vi "Tree.vi"   [LabVIEW 2016, in "LV to ITX.lvclass"]
uses:
  LV to ITX.lvclass
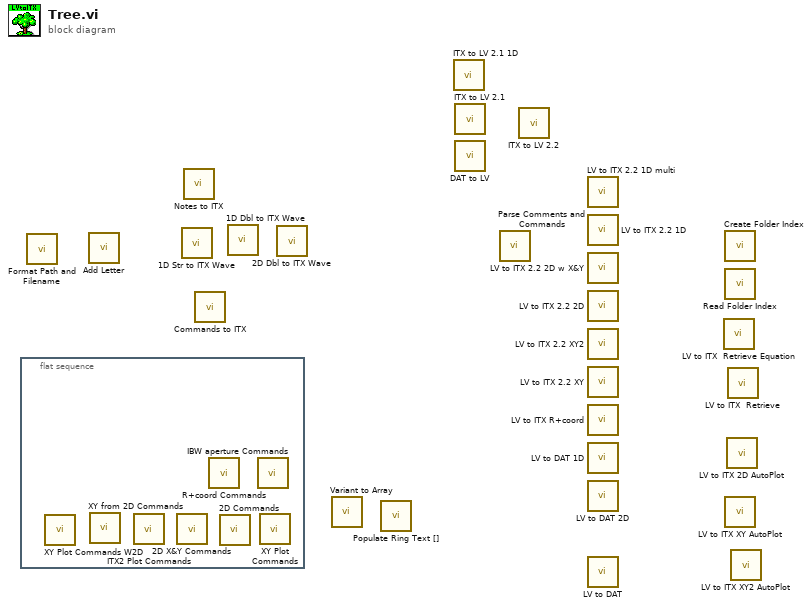
[diagram p0: block diagram]
diagram:
  n1 = flat-sequence {
    frame #0 {
      n2 = call "XY Plot Commands W2D.vi"() -> ()  [unwired: 5 in, 1 out]
      n3 = call "XY from 2D Commands.vi"() -> ()  [unwired: 2 in, 1 out]
      n4 = call "ITX2 Plot Commands.vi"() -> ()  [unwired: 6 in, 1 out]
      n5 = call "2D X&Y Commands.vi"() -> ()  [unwired: 10 in, 2 out]
      n6 = call "R+coord Commands.vi"() -> ()  [unwired: 15 in, 1 out]
      n7 = call "2D Commands.vi"() -> ()  [unwired: 15 in, 1 out]
      n8 = call "IBW aperture Commands.vi"() -> ()  [unwired: 4 in, 1 out]
      n9 = call "XY Plot Commands.vi"() -> ()  [unwired: 6 in, 1 out]
    }
  }
  n10 = call "Format Path and Filename.vi"() -> ()  [unwired: 9 in, 3 out]
  n11 = call "Add Letter.vi"() -> ()  [unwired: 1 in, 1 out]
  n12 = call "1D Str to ITX Wave.vi"() -> ()  [unwired: 2 in, 1 out]
  n13 = call "Notes to ITX.vi"() -> ()  [unwired: 1 in, 1 out]
  n14 = call "Commands to ITX.vi"() -> ()  [unwired: 1 in, 1 out]
  n15 = call "1D Dbl to ITX Wave.vi"() -> ()  [unwired: 2 in, 1 out]
  n16 = call "2D Dbl to ITX Wave.vi"() -> ()  [unwired: 2 in, 1 out]
  n17 = call "Variant to Array.vi"() -> ()  [unwired: 10 in, 2 out]
  n18 = call "Populate Ring Text [].vi"() -> ()  [unwired: 11 in, 1 out]
  n19 = call "ITX to LV 2.1 1D.vi"() -> ()  [unwired: 6 in, 6 out]
  n20 = call "ITX to LV 2.1.vi"() -> ()  [unwired: 6 in, 6 out]
  n21 = call "DAT to LV.vi"() -> ()  [unwired: 7 in, 5 out]
  n22 = call "Parse Comments and Commands.vi"() -> ()  [unwired: 2 in, 2 out]
  n23 = call "ITX to LV 2.2.vi"() -> ()  [unwired: 2 in, 4 out]
  n24 = call "LV to ITX 2.2 1D multi.vi"() -> ()  [unwired: 12 in]
  n25 = call "LV to ITX 2.2 1D.vi"() -> ()  [unwired: 12 in]
  n26 = call "LV to ITX 2.2 2D w X&Y.vi"() -> ()  [unwired: 11 in, 1 out]
  n27 = call "LV to ITX 2.2 2D.vi"() -> ()  [unwired: 12 in]
  n28 = call "LV to ITX 2.2 XY2.vi"() -> ()  [unwired: 11 in, 1 out]
  n29 = call "LV to ITX 2.2 XY.vi"() -> ()  [unwired: 11 in, 1 out]
  n30 = call "LV to ITX R+coord.vi"() -> ()  [unwired: 12 in]
  n31 = call "LV to DAT 1D.vi"() -> ()  [unwired: 10 in, 2 out]
  n32 = call "LV to DAT 2D.vi"() -> ()  [unwired: 10 in, 2 out]
  n33 = call-poly "LV to DAT.vi"() -> ()  [unwired: 10 in, 2 out]
  n34 = call "LV to ITX  Retrieve Equation.vi"() -> ()  [unwired: 11 in, 5 out]
  n35 = call "Create Folder Index.vi"() -> ()  [unwired: 11 in, 1 out]
  n36 = call "Read Folder Index.vi"() -> ()  [unwired: 10 in, 2 out]
  n37 = call "LV to ITX XY AutoPlot.vi"() -> ()  [unwired: 9 in, 3 out]
  n38 = call "LV to ITX 2D AutoPlot.vi"() -> ()  [unwired: 9 in, 3 out]
  n39 = call "LV to ITX  Retrieve.vi"() -> ()  [unwired: 11 in, 5 out]
  n40 = call "LV to ITX XY2 AutoPlot.vi"() -> ()  [unwired: 9 in, 3 out]
